vi "NewCore.vi"(8 "error in":errorcluster, 10 "ParamsArray":variant[](array[variant]), 11 "Pizza":refnum<class "Pizza.lvclass">) -> (0 "error out":errorcluster, 3 "Pizza":refnum<class "Pizza.lvclass">)   [LabVIEW 2020, in "FactoryMethod.lvlib" / "PizzaFactoryMethod.lvlib" / "Pizza.lvclass"]
uses:
  Pizza.lvclass
  Private/TypeDef/privateData.ctl
  TypeDef/PizzaParams.ctl
  Pizza.lvclass/Pizza.ctl
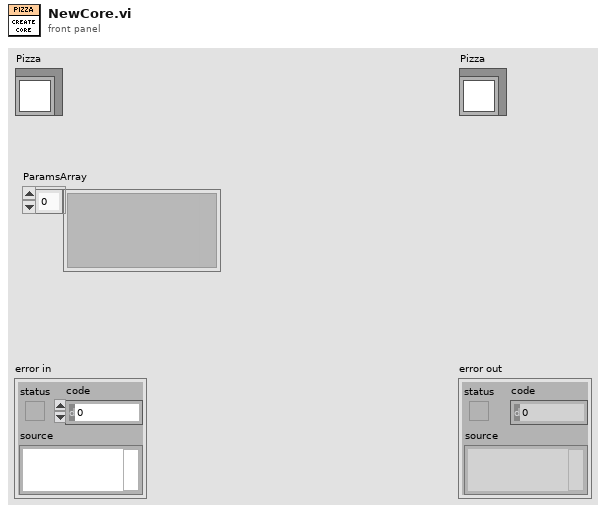
[diagram p1: front panel]
types:
  T1 = typedef "FactoryMethod.lvlib/PizzaFactoryMethod.lvlib/Pizza.lvclass/PizzaParams.ctl" = cluster{"name":string, "dough":string, "sauce":string, "toppings":string[]}
  T2 = typedef "FactoryMethod.lvlib/PizzaFactoryMethod.lvlib/Pizza.lvclass/privateData.ctl" = cluster{"name":string, "dough":string, "sauce":string, "toppings":string[]}
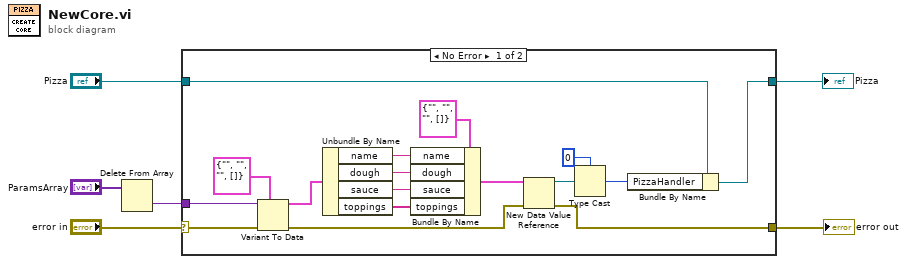
[diagram p0: block diagram]
diagram:
  n1 = Delete From Array(array="ParamsArray") -> (deleted portion=w2:variant)  [unwired: 2 in, 1 out]
  n2 = case shown="No Error" "error in" {
    selector: "error in" -> [w13 w25]
    tunnel: [w16 w25] -> w5
    tunnel: [w18 w24] -> w6
    tunnel: "Pizza" -> [w17 w24]
    tunnel: w2 -> [w11 _]
    frame No Error {
      n3 = Variant To Data(error in=w13, type=T1 {"name"="", "dough"="", "sauce"="", "toppings"=[]} ("<ClassName>Params"), Variant=w11) -> (data=w14:T1, error out=w12:errorcluster)
      n4 = Unbundle By Name(w14) -> ("name"=w10:string, "dough"=w9:string, "sauce"=w8:string, "toppings"=w7:string[])
      n5 = Bundle By Name(cluster=T2 {"name"="", "dough"="", "sauce"="", "toppings"=[]} ("privateData"), "name"=w10, "dough"=w9, "sauce"=w8, "toppings"=w7) -> (w19:T2)
      n6 = New Data Value Reference(data value=w19, error in=w12) -> (data value reference=w23:refnum<data-value>, error out=w16:errorcluster)
      n7 = Type Cast(type=u32 0, x=w23) -> (*(type *) &x=w21:u32)
      n8 = Bundle By Name(cluster=w17, "PizzaHandler"=w21) -> (w18:refnum<class "Pizza.lvclass">)
    }
    frame Error {
    }
  }
  "error out" <- w5
  "Pizza" <- w6
